vi "Configure Output Timer.vi"(6 "Enable Output Timer (T: Enable)":bool=TRUE, 7 "Channel Select":enum16{"Channel 1", "Channel 2", "Channel 3"}(ring), 8 "error in (no error)":errorcluster, 9 "Enable Output (T: Enable)":bool=TRUE, 10 "Output Timer(0)":dbl format="%#_2g", 11 "VISA resource name":refnum<visa-resource-name>) -> (0 "error out":errorcluster, 3 "VISA resource name out":refnum<visa-resource-name>)   [LabVIEW 2018, in "Keithley KE22xx Series.lvlib"]
doc: "Configure the output-timer, select the desired Channel and,\nTo start Timer \n- First, set OUTPUT:TIMER ON, then set OUTPUT ON. \nTo end Timer \n- Set OUTPUT:TIMER OFF to turn timer off."
uses:
  Keithley KE22xx Series.lvlib
panel:
  # "© 2012 Keithley Instruments, Inc. ALL RIGHTS RESERVED"
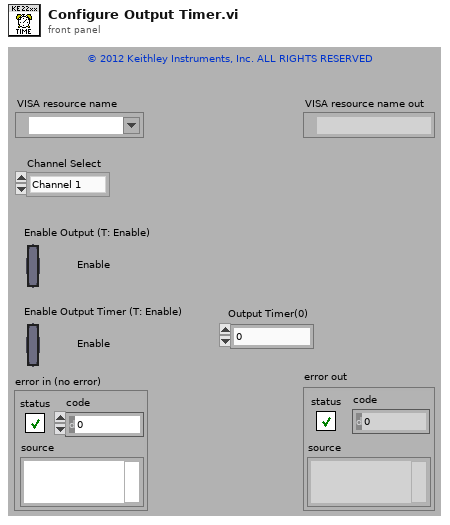
[diagram p1: front panel]
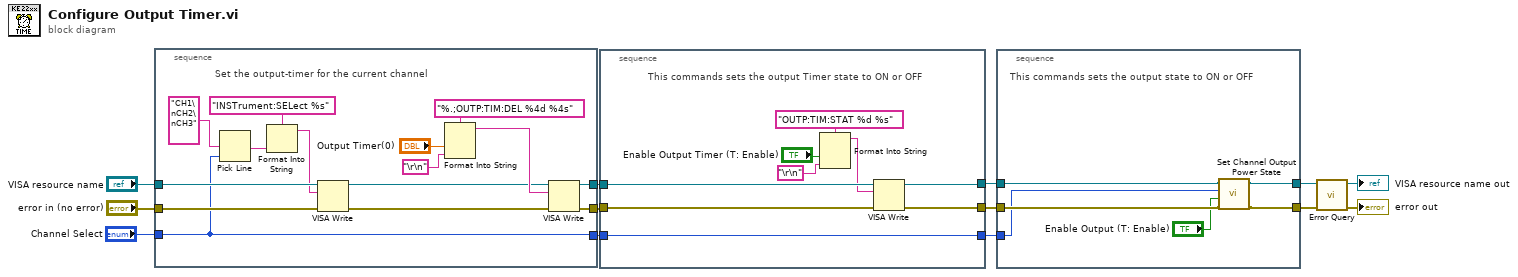
[diagram p0: block diagram]
diagram:
  n1 = stacked-sequence {
    tunnel: "VISA resource name" -> [w19]
    tunnel: "error in (no error)" -> [w18]
    tunnel: [w24] -> w9
    tunnel: [w23] -> w8
    tunnel: "Channel Select" -> [w14]
    tunnel: [w14] -> w2
    frame #0 {
      # "Set the output-timer for the current channel"
      n2 = Pick Line(multi-line string="CH1\nCH2\nCH3", line index=w14) -> (output string=w22:string)  [unwired: 1 in]
      n3 = Format Into String(format string="INSTrument:SELect %s", w22) -> (resulting string=w15:string)  [unwired: 2 in, 1 out]
      n4 = VISA Write(VISA resource name=w19, write buffer=w15, error in (no error)=w18) -> (VISA resource name out=w16:refnum<visa-resource-name>, error out=w17:errorcluster)  [unwired: 1 out]
      n5 = Format Into String(format string="%.;OUTP:TIM:DEL %4d %4s", "Output Timer(0)", "\r\n") -> (resulting string=w26:string)  [unwired: 2 in, 1 out]
      n6 = VISA Write(VISA resource name=w16, write buffer=w26, error in (no error)=w17) -> (VISA resource name out=w24:refnum<visa-resource-name>, error out=w23:errorcluster)  [unwired: 1 out]
    }
  }
  n7 = stacked-sequence {
    tunnel: w9 -> [w35]
    tunnel: w8 -> [w34]
    tunnel: [w33] -> w7
    tunnel: [w32] -> w6
    tunnel: w2 -> [w29]
    tunnel: [w29] -> w1
    frame #0 {
      # "This commands sets the output Timer state to ON or OFF"
      n8 = Format Into String(format string="OUTP:TIM:STAT %d %s", "Enable Output Timer (T: Enable)", "\r\n") -> (resulting string=w31:string)  [unwired: 2 in, 1 out]
      n9 = VISA Write(VISA resource name=w35, write buffer=w31, error in (no error)=w34) -> (VISA resource name out=w33:refnum<visa-resource-name>, error out=w32:errorcluster)  [unwired: 1 out]
    }
  }
  n10 = stacked-sequence {
    tunnel: w7 -> [w43]
    tunnel: w6 -> [w41]
    tunnel: [w42] -> w5
    tunnel: [w40] -> w4
    tunnel: w1 -> [w39]
    frame #0 {
      # "This commands sets the output state to ON or OFF"
      n11 = call "Set Channel Output Power State.vi"("error in (no error)"=w41, "Enable Output (T: On)"="Enable Output (T: Enable)", "Channel Select"=w39, "Visa Resource Name IN"=w43) -> ("error out"=w40:errorcluster, "Visa Resource Name OUT"=w42:refnum<visa-resource-name>)  [unwired: 6 in]
    }
  }
  n12 = call "Error Query.vi"("error in (no error)"=w4, "VISA resource name"=w5) -> ("error out"=→"error out":errorcluster, "VISA resource name out"=→"VISA resource name out":refnum<visa-resource-name>)  [unwired: 6 in, 2 out]
